vi "Teleop.vi"(10 "Match Info":T1={"Autonomous Elapsed Seconds"=0.0, "TeleOp Elapsed Seconds"=0.0, "Disabled Elapsed Seconds"=0.0, "Visited Autonomous"=FALSE, "Visited TeleOp"=FALSE, "Visited Disabled"=FALSE, "Autonomous Settings"={"Autonomous Style"=enum."Independent", "VI Refnum"=refnum}}, 11 "Call Context":T2) -> ()   [LabVIEW 2015]
doc: "This VI is called for each TeleOp packet received from the DS where the robot is not disabled. It is often used to read from the joysticks and update I/O or to update setpoints for timed control loops. It should complete and return within 20 milliseconds or it may miss DS packets."
uses:
  <vilib>/Rock Robotics/WPI/DriverStation/WPI_DriverStationDerivedRobotMode.ctl
  <vilib>/Rock Robotics/WPI/DriverStation/WPI_DriverStationMatch Info.ctl
  <vilib>/Rock Robotics/WPI/CAN/TalonSRX/WPI_CANTalonSRX_APIControlMode.ctl
  <vilib>/Rock Robotics/WPI/Solenoid/WPI_SolenoidValue.ctl
  <vilib>/Rock Robotics/WPI/Utilities/WPI_GetSetVariantRefNum.vi
  <vilib>/Rock Robotics/Network Tables/NT Read Number.vi
  <vilib>/Rock Robotics/Network Tables/NT Write Boolean.vi
  <vilib>/Rock Robotics/WPI/Solenoid/WPI_SolenoidSetEnum.vi
  <vilib>/Rock Robotics/Network Tables/NT Write Number.vi
  <vilib>/addons/control/pid/NI_PID_pid.lvlib
  <vilib>/addons/control/pid/pid.llb/PID (DBL).vi
  <vilib>/Rock Robotics/WPI/Ultrasonic/WPI_SonarMB1010AnalogRefNum Registry Get.vi
  <vilib>/Rock Robotics/WPI/Ultrasonic/WPI_SonarMB1010AnalogGetRange.vi
panel:
  out "right encoder":dbl
  out "left encoder":dbl
  out "Numeric":dbl
  out "Angular Rate":dbl
  out "Angle":dbl
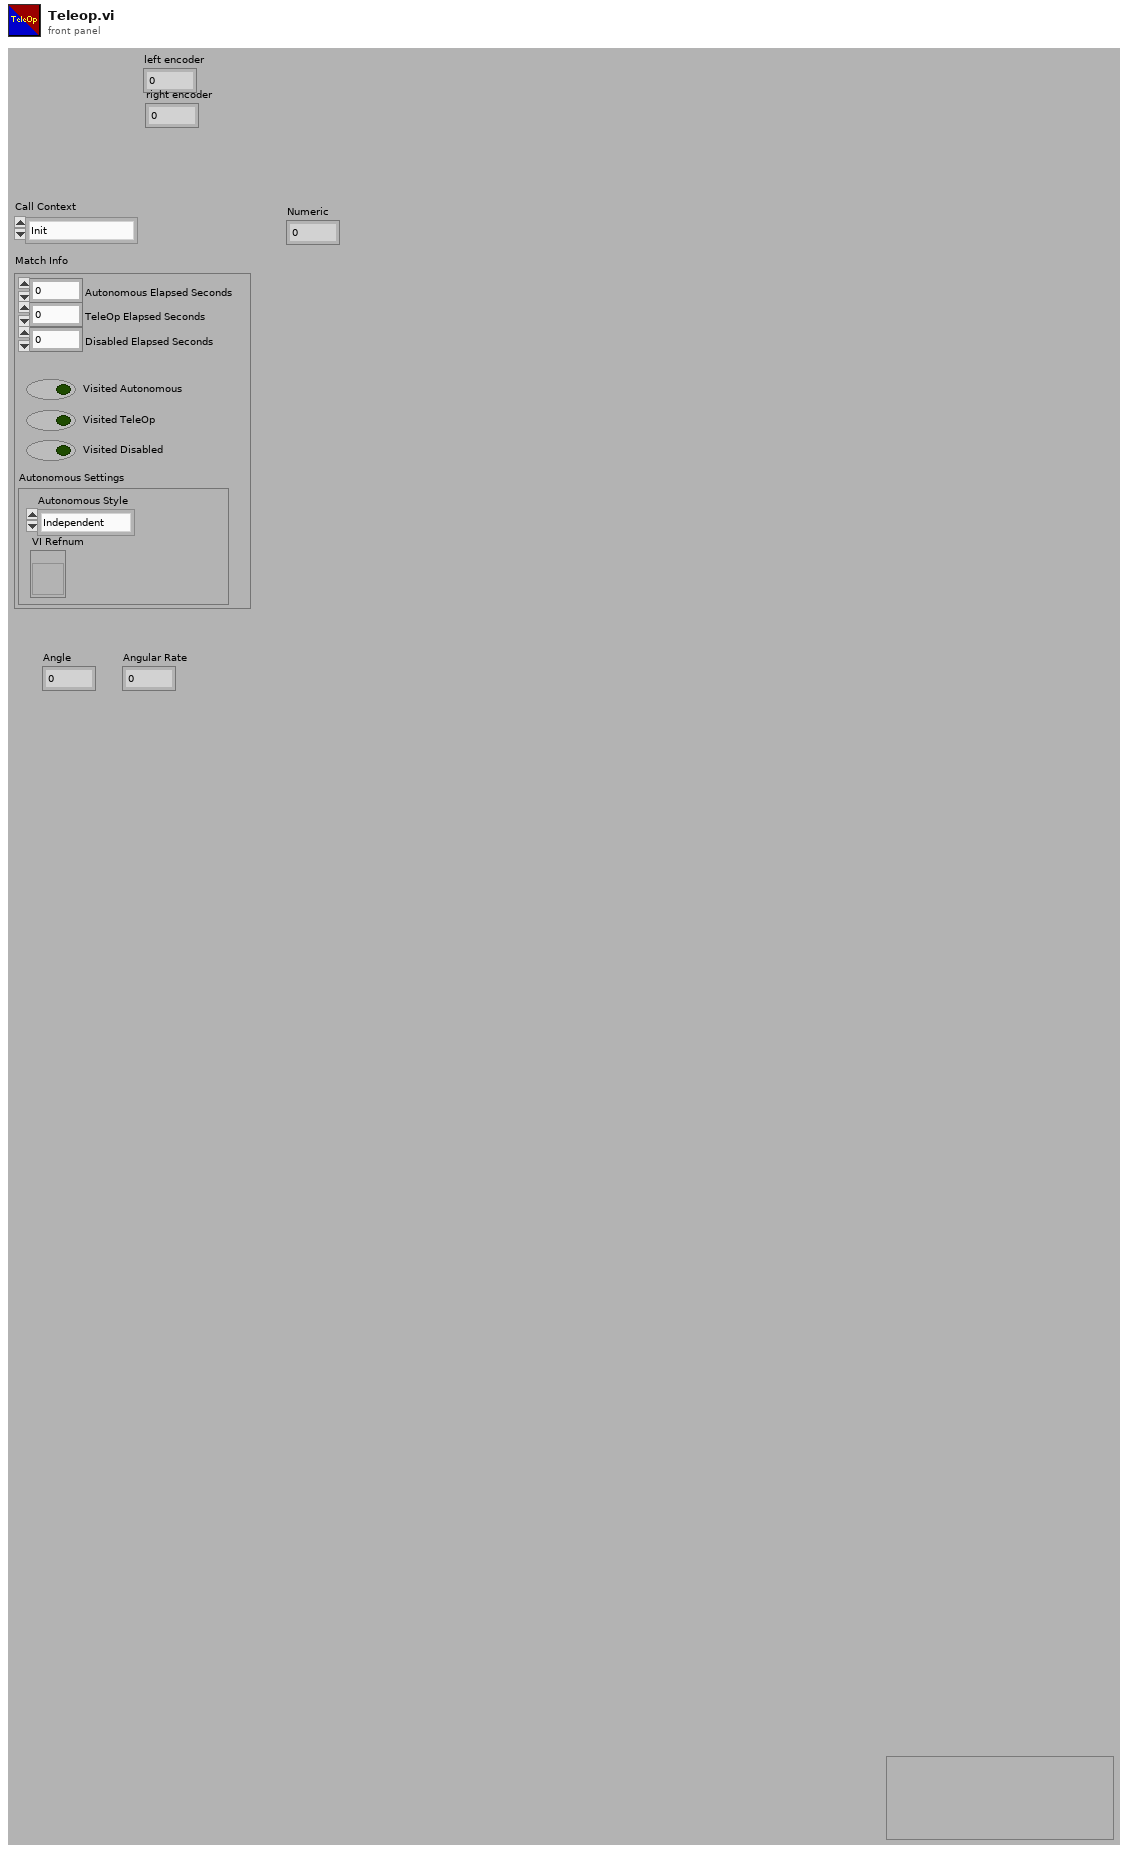
[diagram p1: front panel]
types:
  T1 = typedef "WPI_DriverStationMatch Info.ctl" = cluster{"Autonomous Elapsed Seconds":dbl, "TeleOp Elapsed Seconds":dbl, "Disabled Elapsed Seconds":dbl, "Visited Autonomous":bool, "Visited TeleOp":bool, "Visited Disabled":bool, "Autonomous Settings":cluster{"Autonomous Style":enum16{"Iterative", "Independent"}, "VI Refnum":refnum<vi>}}
  T2 = typedef "WPI_DriverStationDerivedRobotMode.ctl" = enum16{"Init", "Execute", "Stop"}
  T3 = typedef "WPI_JoystickDevRef.ctl" = cluster{"Device":T4}
  T4 = typedef "WPI_JoystickDeviceEnum.ctl" = enum16{"USB 0", "USB 1", "USB 2", "USB 3", "USB 4", "USB 5"}
  T5 = typedef "WPI_CANTalonSRX_APIControlMode.ctl" = enum8{"Percent VBus", "Speed", "Position", "Slave", "Unchanged / Invalid", "Voltage Compensation", "Current", "Motion Profile"}
  T6 = typedef "WPI_SolenoidValue.ctl" = enum16{"Off", "On", "Forward", "Reverse"}
  T7 = typedef "WPI_GyroDevRef.ctl" = cluster{"DevStatus":errorcluster, "Analog Channel":T8, "Offset":dbl, "Gain (VoltsPerDegree/Second)":dbl, "Gyro Type":enum16{"Analog", "XRS450"}, "Handle":i32, "SPI Bus":T9, "Device Found":bool, "Sample Rate":dbl, "Calibrate On Open":bool}
  T8 = typedef "FPGA_AIChannel.ctl" = enum8{"AI 0", "AI 1", "AI 2", "AI 3", "AI MXP 0", "AI MXP 1", "AI MXP 2", "AI MXP 3", "Invalid"}
  T9 = typedef "spi_bus.ctl" = enum16{"SPI On-Board, CS0", "SPI On-Board, CS1", "SPI On-Board, CS2", "SPI On-Board, CS3", "SPI MXP", "Invalid"}
  T10 = typedef "WPI_MotorControlDeviceRef.ctl" = cluster{"DeviceStatus":errorcluster, "Type":T11, "PWM":cluster{"PWM Channel":T12, "DeadBand":T13}, "CAN":cluster{"Device Number":u8, "Control Mode":T14, "Semaphore":T15, "Max Vout":dbl, "TalonSRX Control Mode":T5}, "Invert":bool}
  T11 = typedef "WPI_MotorControlType.ctl" = enum16{"PWM", "CAN", "CANTalonSRX"}
  T12 = typedef "FPGA_DIOPWMChannel.ctl" = enum8{"PWM 0", "PWM 1", "PWM 2", "PWM 3", "PWM 4", "PWM 5", "PWM 6", "PWM 7", "PWM 8", "PWM 9", "PWM MXP 0", "PWM MXP 1", "PWM MXP 2", "PWM MXP 3", "PWM MXP 4", "PWM MXP 5", "PWM MXP 6", "PWM MXP 7", "PWM MXP 8", "PWM MXP 9", "Invalid"}
  T13 = typedef "WPI_PWMDeadband.ctl" = cluster{"Name":string, "maxPositivePwm":i32, "minPositivePwm":i32, "centerPwm":i32, "maxNegativePwm":i32, "minNegativePwm":i32, "angularRange":u16}
  T14 = typedef "WPI_CANJaguar_ControlMode.ctl" = enum8{"Percent VBus", "Current", "Speed", "Position", "Voltage"}
  T15 = typedef "Semaphore RefNum" = refnum<k1>
  T16 = typedef "WPI_ServoDeviceRef.ctl" = cluster{"DeviceStatus":errorcluster, "PWM Channel":T12, "DeadBand":T13}
  T17 = typedef "WPI_CANTalonSRX_GlobalStatus.ctl" = cluster{"Applied Throttle":dbl, "Module Enabled":bool, "CAN Error":errorcluster, "Closed Loop Error":dbl, "Forward Limit Switch Closed":bool, "Reverse Limit Switch Closed":bool, "Sensor Position":dbl, "Sensor Velocity":dbl, "Current":dbl, "Sticky Fault - Over Temp":bool, "Sticky Fault - Under Voltage":bool, "Sticky Fault - Forward Limit":bool, "Sticky Fault - Reverse Limit":bool, "Sticky Fault - Forward Soft Limit":bool, "Sticky Fault - Reverse Soft Limit":bool, "Brake is Enabled":bool, "Encoder Position":dbl, "Encoder Velocity":dbl, "Encoder Index Count":dbl, "Encoder A Pin State":bool, "Encoder B Pin State":bool, "Encoder Index Pin State":bool, "Analog In":dbl, "Analog In Velocity":dbl, "Temperature (C)":dbl, "Battery Voltage":dbl, "Control 5 Is Supported":bool, "Current Profile Slot Select":dbl, "Pos Div 8":bool, "Vel Div 4":bool, "Pulse Width Position":i32, "Pulse Width Velocity":i32, "Pulse Width Rise To Rise (us)":i32, "Pulse Width Rise To Fall (us)":i32, "Mot Prof Active Is Under Run":bool, "Mot Prof Active Has Under Run":bool, "Mot Prof Active Is Last":bool, "Mot Prof Active Velocity Only":bool, "Mot Prof Active Is Valid":bool, "Mot Prof Buffer Is Full":bool, "Mot Prof Active Profile Slot Select":i32, "Mot Prof NextID":i32, "Mot Prof Count":i32, "Mot Prof Active Velocity":dbl, "Mot Prof Active Position":dbl, "Mot Prof Output Enable":i32}
  T18 = typedef "WPI_SonarMB1010AnalogDeviceRef.ctl" = cluster{"AIDeviceRef":T19, "Scaling factor (V/in)":dbl, "Average Bits":u8}
  T19 = typedef "WPI_AnalogChannelDevRef.ctl" = cluster{"DevStatus":errorcluster, "Analog Channel":T8}
  T20 = typedef "WPI_SolenoidDevRef.ctl" = cluster{"DevStatus":errorcluster, "Pneumatics Control Module":u8, "Forward Solenoid Channel":T21, "Reverse Solenoid Channel":T21}
  T21 = typedef "WPI_SolenoidChannel.ctl" = enum8{"Solenoid 0", "Solenoid 1", "Solenoid 2", "Solenoid 3", "Solenoid 4", "Solenoid 5", "Solenoid 6", "Solenoid 7", "Invalid"}
  T22 = cluster{"proportional gain (Kc)":dbl, "integral time (Ti, min)":dbl, "derivative time (Td, min)":dbl}
  T23 = typedef "WPI_PotentiometerDevRef.ctl" = cluster{"DevStatus":errorcluster, "Analog Channel":T8, "Invert Output":bool}
  T24 = cluster{"Aiming?":bool, "X setpoint":dbl, "Y-setpoint":dbl}
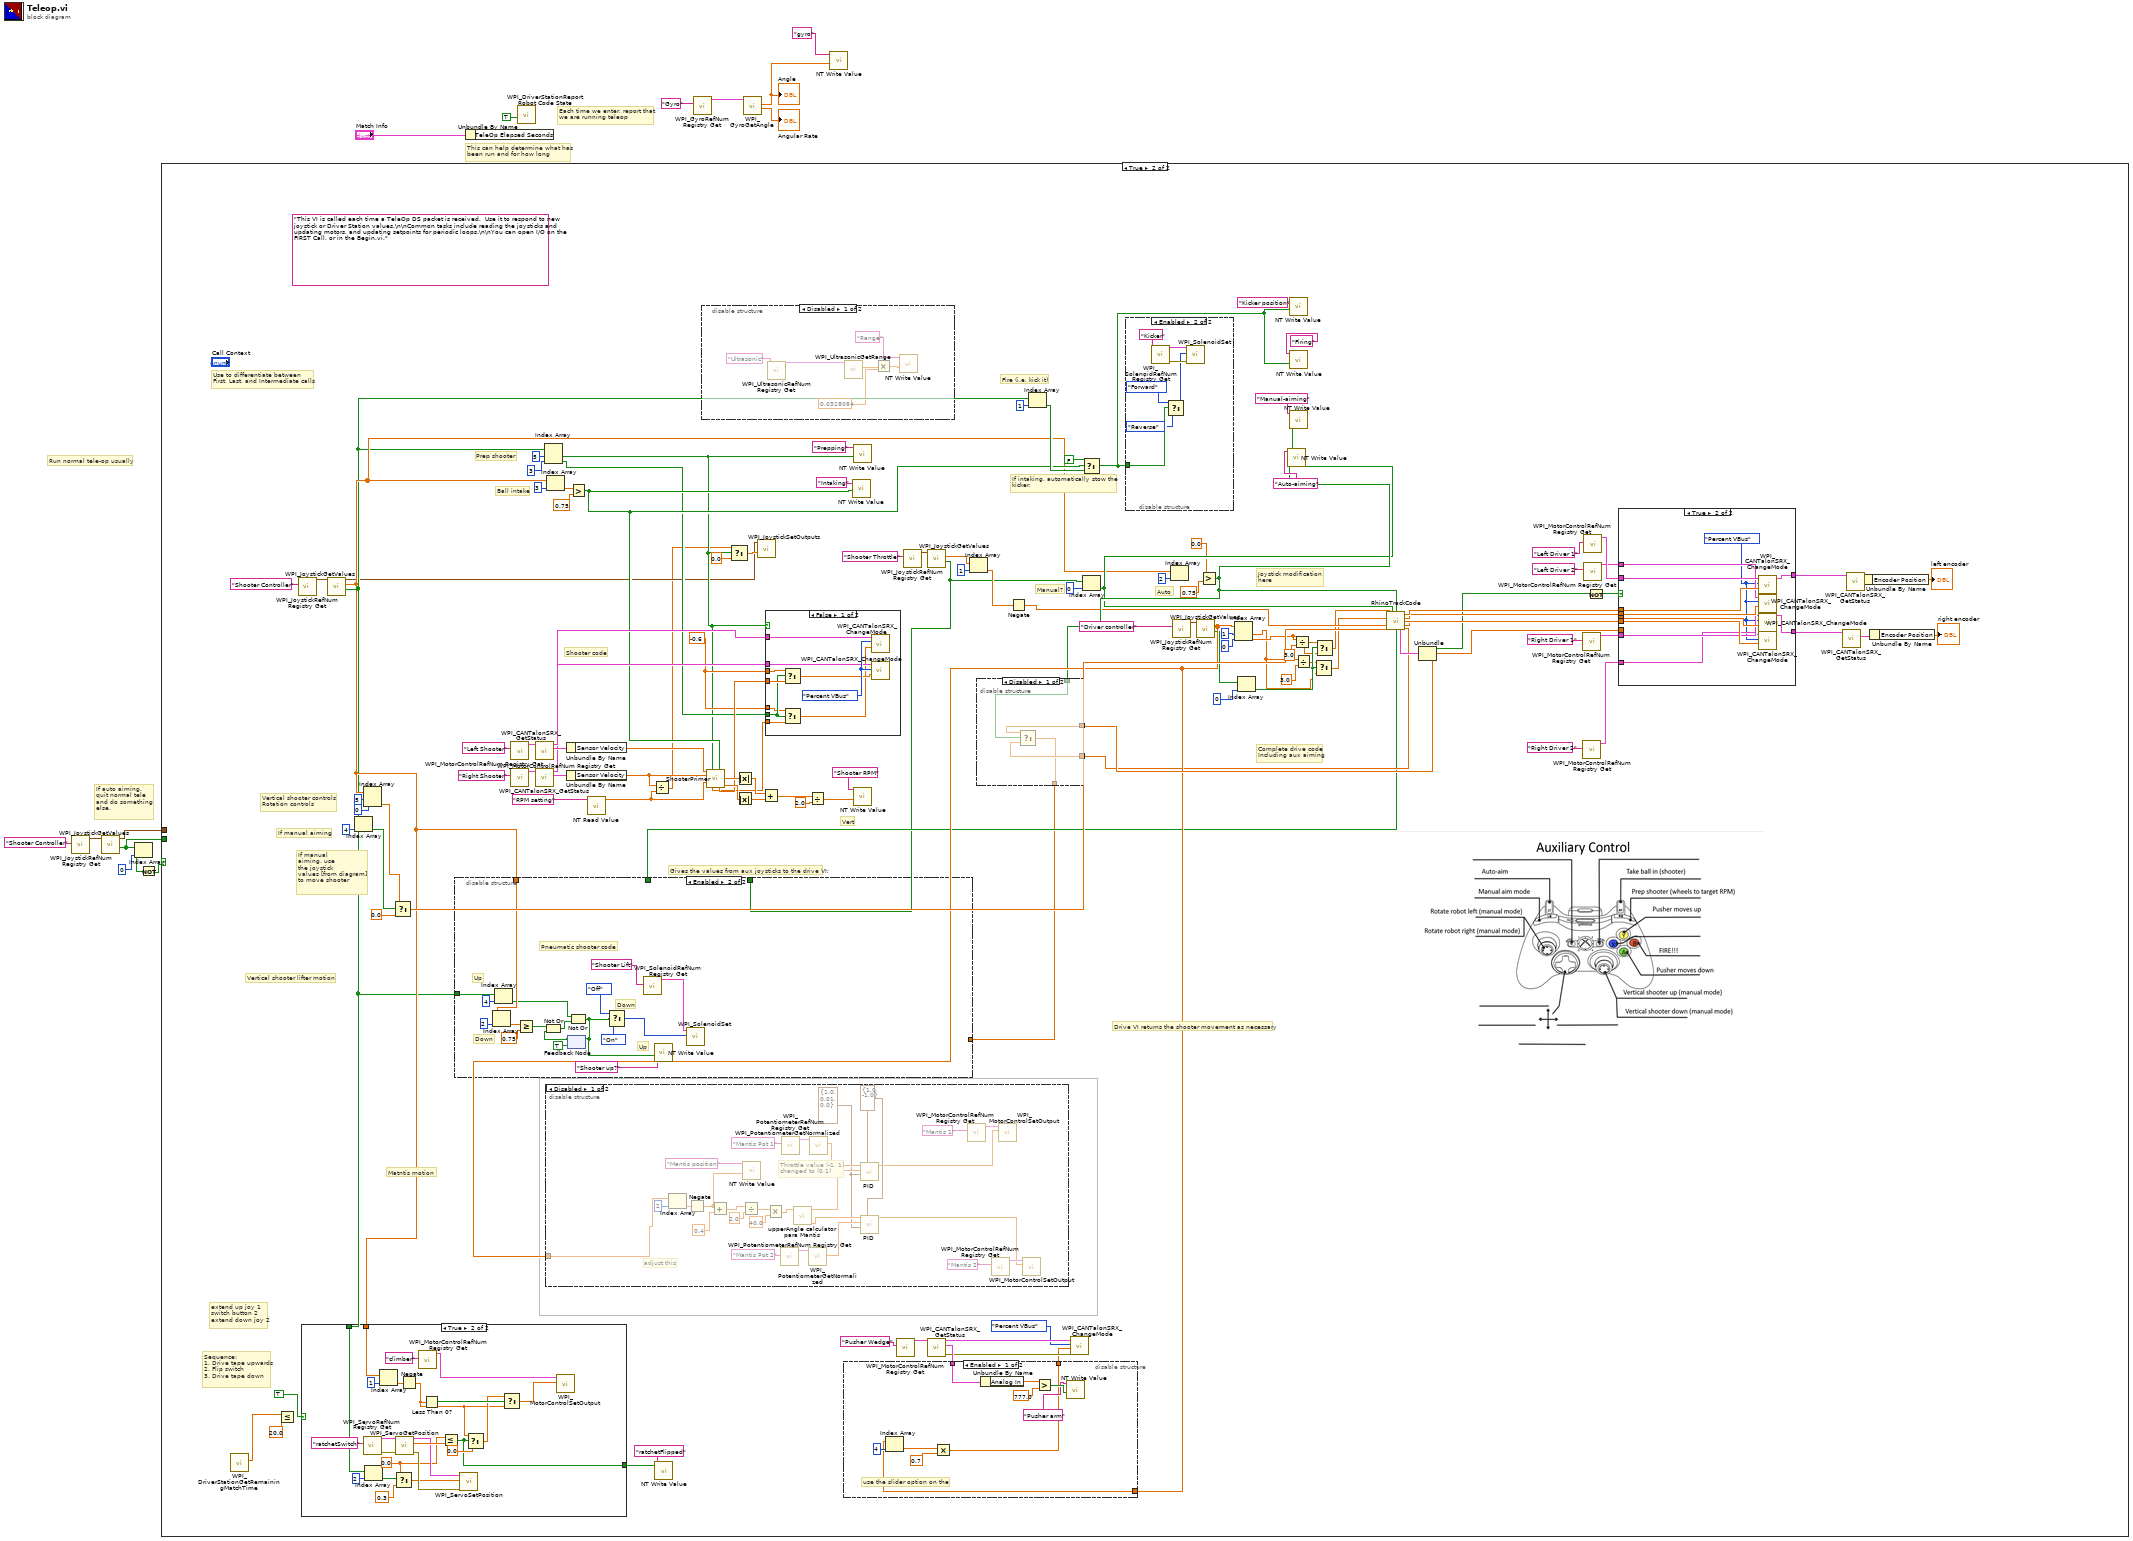
[diagram p0: block diagram]
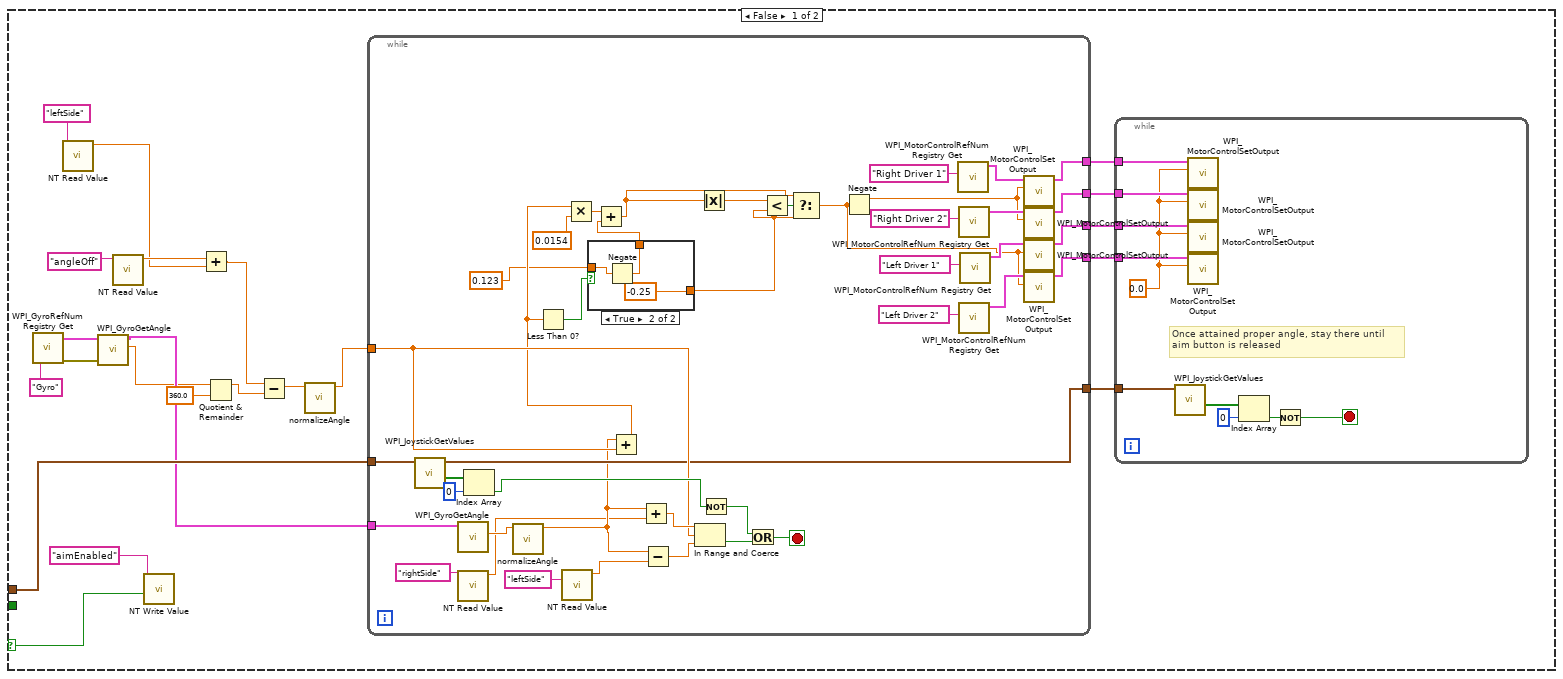
[diagram p2: hidden frame]
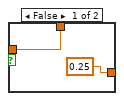
[diagram p3: hidden frame]
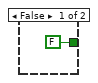
[diagram p4: hidden frame]
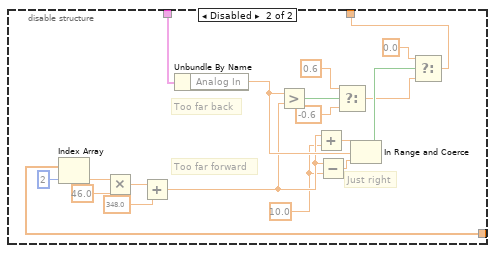
[diagram p5: hidden frame]
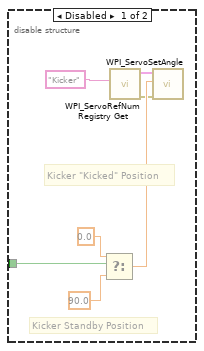
[diagram p6: hidden frame]
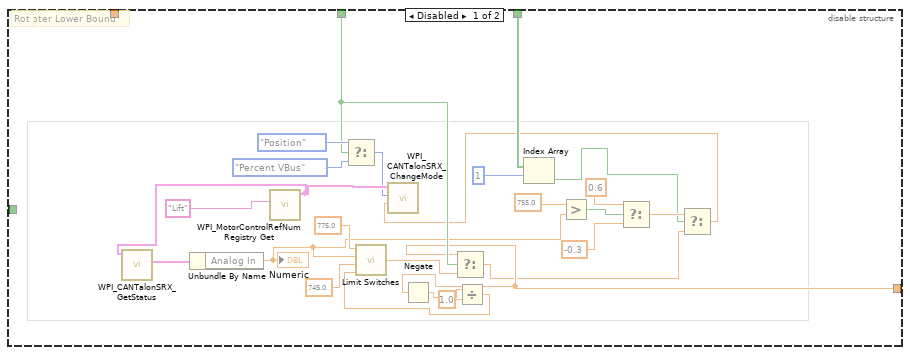
[diagram p8: hidden frame]
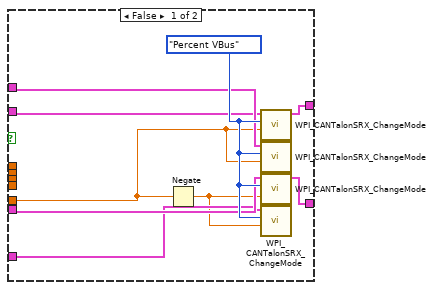
[diagram p10: hidden frame]
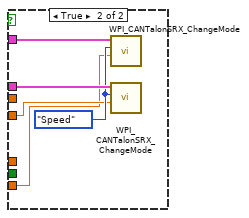
[diagram p11: hidden frame]
diagram:
  # "If auto aiming,\nquit normal tele\nand do something\nelse,"
  # "Run normal tele-op usually"
  # "This can help determine what has\nbeen run and for how long"
  # "Each time we enter, report that\nwe are running teleop"
  n1 = call <vilib>:"WPI_JoystickRefNum Registry Get.vi"("refnum name"="Shooter Controller") -> ("JoystickDevRef"=w11:T3)  [unwired: 9 in, 1 out]
  n2 = call <vilib>:"WPI_JoystickGetValues.vi"("JoystickDevRef"=w11) -> ("Buttons"=w8:bool[], "JoystickDevRef"=w1:T3)  [unwired: 6 in, 3 out]
  n3 = Index Array(array=w8, index=0) -> (element=w9:bool)
  n4 = Not(x=w9) -> (.not. x?=w7:bool)
  n5 = case shown="True" w7 {
    selector: w7 -> [w35 _]
    tunnel: w8 -> [_ _]
    tunnel: w1 -> [w33 _]
    frame False {
      n6 = call <vilib>:"WPI_GyroRefNum Registry Get.vi"("refnum name"="Gyro") -> ("error out"=w24:errorcluster, "GyroDevRef"=w25:T7)  [unwired: 9 in]
      n7 = call-poly <vilib>:"NT Read Value.vi"("Name"="leftSide") -> ("Numeric"=w16:dbl)  [unwired: 9 in, 1 out]
      n8 = call <vilib>:"WPI_GyroGetAngle.vi"("error in"=w24, "GyroDevRef"=w25) -> ("Angle"=w23:dbl, "GyroDevRef"=w26:T7)  [unwired: 5 in, 3 out]
      n9 = call-poly <vilib>:"NT Read Value.vi"("Name"="angleOff") -> ("Numeric"=w18:dbl)  [unwired: 9 in, 1 out]
      n10 = call-poly <vilib>:"NT Write Value.vi"("Boolean"=w35, "Name"="aimEnabled") -> ()  [unwired: 9 in, 1 out]
      n11 = Add(x=w18, y=w16) -> (x+y=w17:dbl)
      n12 = Quotient & Remainder(x=w23, y=360.0) -> (x-y*floor(x/y)=w21:dbl)  [unwired: 1 out]
      n13 = Subtract(x=w17, y=w21) -> (x-y=w20:dbl)
      n14 = call "normalizeAngle.vi"("Input"=w20) -> ("Output"=w19:dbl)  [unwired: 10 in]
      n15 = while {
        tunnel: w33 -> [w80]
        tunnel: w26 -> [w77]
        tunnel: w19 -> [w70]
        tunnel: [w69] -> w31
        tunnel: [w68] -> w30
        tunnel: [w67] -> w29
        tunnel: [w66] -> w28
        tunnel: [w65] -> w27
        stop <- w71 stop-if-true
        n16 = call <vilib>:"WPI_JoystickGetValues.vi"("JoystickDevRef"=w80) -> ("Buttons"=w79:bool[], "JoystickDevRef"=w65:T3)  [unwired: 6 in, 3 out]
        n17 = call <vilib>:"WPI_GyroGetAngle.vi"("GyroDevRef"=w77) -> ("Angle"=w62:dbl)  [unwired: 6 in, 4 out]
        n18 = call-poly <vilib>:"NT Read Value.vi"("Name"="rightSide") -> ("Numeric"=w49:dbl)  [unwired: 9 in, 1 out]
        n19 = Index Array(array=w79, index=0) -> (element=w72:bool)
        n20 = call "normalizeAngle.vi"("Input"=w62) -> ("Output"=w61:dbl)  [unwired: 10 in]
        n21 = call-poly <vilib>:"NT Read Value.vi"("Name"="leftSide") -> ("Numeric"=w50:dbl)  [unwired: 9 in, 1 out]
        n22 = Add(x=w61, y=w70) -> (x+y=w60:dbl)
        n23 = Less Than 0?(x=w60) -> (x < 0?=w54:bool)
        n24 = Multiply(x=w60, y=0.0154) -> (x*y=w58:dbl)
        n25 = case shown="True" w54 {
          tunnel: 0.123 ("y") -> [w90 w93]
          tunnel: [w90 w92] -> w52
          tunnel: [0.25 ("y") -0.25 ("y")] -> w51
          frame False {
          }
          frame True {
            n26 = Negate(x=w93) -> (-x=w92:dbl)
          }
        }
        n27 = Add(x=w58, y=w52) -> (x+y=w56:dbl)
        n28 = Add(x=w61, y=w49) -> (x+y=w76:dbl)
        n29 = Subtract(x=w61, y=w50) -> (x-y=w75:dbl)
        n30 = In Range and Coerce(upper limit=w76, x=w70, lower limit=w75) -> (In Range?=w74:bool)  [unwired: 1 out]
        n31 = Absolute Value(x=w56) -> (abs(x)=w55:dbl)
        n32 = Not(x=w72) -> (.not. x?=w73:bool)
        n33 = Or(x=w73, y=w74) -> (x .or. y?=w71:bool)
        n34 = Less?(x=w55, y=w51) -> (x < y?=w57:bool)
        n35 = Select(t=w56, s=w57, f=w51) -> (s? t:f=w64:dbl)
        n36 = Negate(x=w64) -> (-x=w63:dbl)
        n37 = call <vilib>:"WPI_MotorControlRefNum Registry Get.vi"("refnum name"="Right Driver 1") -> ("MotorControlDevRef"=w84:T10)  [unwired: 9 in, 1 out]
        n38 = call <vilib>:"WPI_MotorControlRefNum Registry Get.vi"("refnum name"="Right Driver 2") -> ("MotorControlDevRef"=w83:T10)  [unwired: 9 in, 1 out]
        n39 = call <vilib>:"WPI_MotorControlRefNum Registry Get.vi"("refnum name"="Left Driver 2") -> ("MotorControlDevRef"=w81:T10)  [unwired: 9 in, 1 out]
        n40 = call <vilib>:"WPI_MotorControlRefNum Registry Get.vi"("refnum name"="Left Driver 1") -> ("MotorControlDevRef"=w82:T10)  [unwired: 9 in, 1 out]
        n41 = call <vilib>:"WPI_MotorControlSetOutput.vi"("Output"=w63, "MotorControlDevRef"=w84) -> ("MotorControlDevRef"=w69:T10)  [unwired: 7 in, 2 out]
        n42 = call <vilib>:"WPI_MotorControlSetOutput.vi"("Output"=w63, "MotorControlDevRef"=w83) -> ("MotorControlDevRef"=w68:T10)  [unwired: 7 in, 2 out]
        n43 = call <vilib>:"WPI_MotorControlSetOutput.vi"("Output"=w64, "MotorControlDevRef"=w82) -> ("MotorControlDevRef"=w67:T10)  [unwired: 7 in, 2 out]
        n44 = call <vilib>:"WPI_MotorControlSetOutput.vi"("Output"=w64, "MotorControlDevRef"=w81) -> ("MotorControlDevRef"=w66:T10)  [unwired: 7 in, 2 out]
      }
      n45 = while {
        tunnel: w31 -> [w46]
        tunnel: w30 -> [w45]
        tunnel: w29 -> [w44]
        tunnel: w28 -> [w43]
        tunnel: w27 -> [w41]
        stop <- w37 stop-if-true
        w42 = 0.0
        # "Once attained proper angle, stay there until \naim button is released"
        n46 = call <vilib>:"WPI_JoystickGetValues.vi"("JoystickDevRef"=w41) -> ("Buttons"=w40:bool[])  [unwired: 6 in, 4 out]
        n47 = call <vilib>:"WPI_MotorControlSetOutput.vi"("Output"=w42, "MotorControlDevRef"=w46) -> ()  [unwired: 7 in, 3 out]
        n48 = call <vilib>:"WPI_MotorControlSetOutput.vi"("Output"=w42, "MotorControlDevRef"=w45) -> ()  [unwired: 7 in, 3 out]
        n49 = call <vilib>:"WPI_MotorControlSetOutput.vi"("Output"=w42, "MotorControlDevRef"=w44) -> ()  [unwired: 7 in, 3 out]
        n50 = call <vilib>:"WPI_MotorControlSetOutput.vi"("Output"=w42, "MotorControlDevRef"=w43) -> ()  [unwired: 7 in, 3 out]
        n51 = Index Array(array=w40, index=0) -> (element=w38:bool)
        n52 = Not(x=w38) -> (.not. x?=w37:bool)
      }
    }
    frame True {
      w127 = -0.6
      (unwired) "This VI is called each time a TeleOp DS packet is received.  Use it to respond to new joystick or Driver Station values.\n\nCommon tasks include reading the joysticks and updating motors, and updating setpoints for periodic loops.\n\nYou can open I/O on the FIRST Call, or in the Begin.vi."
      # "extend up joy 1\nswitch button 2\nextend down joy 2"
      # "Sequence:\n1. Drive tape upwards\n2. Flip switch\n3. Drive tape down"
      # "Auto"
      # "Manual?"
      # "Joystick modification\nhere"
      # "Complete drive code\nIncluding aux aiming"
      # "If intaking, automatically stow the\nkicker,"
      # "Fire (i.e, kick it)"
      # "Shooter code"
      # "Drive VI returns the shooter movement as necessary"
      # "Gives the values from aux joysticks to the drive VI;"
      # "Vert"
      # "If manual \naiming, use\nthe joystick\nvalues [from diagram]\nto move shooter"
      # "Vertical shooter controls\nRotation controls"
      # "If manual aiming"
      # "Ball intake"
      # "Prep shooter"
      # "Matntis motion"
      # "Vertical shooter lifter motion"
      # "Use to differentiate between\nFirst, Last, and Intermediate calls"
      n53 = call <vilib>:"WPI_DriverStationGetRemainingMatchTime.vi"() -> ("Match Time(s)"=w110:sgl)  [unwired: 10 in, 1 out]
      n54 = Less Or Equal?(x=w110, y=20.0) -> ()  [unwired: 1 out]
      n55 = call <vilib>:"WPI_JoystickRefNum Registry Get.vi"("refnum name"="Shooter Controller") -> ("JoystickDevRef"=w215:T3)  [unwired: 9 in, 1 out]
      n56 = call <vilib>:"WPI_JoystickGetValues.vi"("JoystickDevRef"=w215) -> ("Buttons"=w112:bool[], "Axes"=w113:dbl[], "JoystickDevRef"=w103:T3)  [unwired: 6 in, 2 out]
      n57 = case shown="True" TRUE {
        tunnel: w113 -> [_ w240]
        tunnel: w112 -> [_ w239]
        tunnel: [FALSE w218] -> w108
        frame False {
        }
        frame True {
          w219 = 0.0 ("t")
          n58 = call <vilib>:"WPI_ServoRefNum Registry Get.vi"("refnum name"="ratchetSwitch") -> ("error out"=w232:errorcluster, "ServoDeviceRef"=w233:T16)  [unwired: 9 in]
          n59 = Index Array(array=w239, index=2) -> (element=w221:bool)
          n60 = Index Array(array=w240, index=1) -> (element=w230:dbl)
          n61 = Select(t=w219, s=w221, f=0.3) -> (s? t:f=w222:dbl)
          n62 = call <vilib>:"WPI_ServoGetPosition.vi"("error in (no error)"=w232, "ServoDeviceRef"=w233) -> ("error out"=w223:errorcluster, "Position"=w229:dbl, "ServoDeviceRef"=w224:T16)  [unwired: 7 in]
          n63 = Negate(x=w230) -> (-x=w226:dbl)
          n64 = call <vilib>:"WPI_MotorControlRefNum Registry Get.vi"("refnum name"="climber") -> ("MotorControlDevRef"=w234:T10)  [unwired: 9 in, 1 out]
          n65 = Less Than 0?(x=w226) -> (x < 0?=w231:bool)
          n66 = Less Or Equal?(x=w219, y=w229) -> (x <= y?=w218:bool)
          n67 = call <vilib>:"WPI_ServoSetPosition.vi"("error in (no error)"=w223, "Position"=w222, "ServoDeviceRef"=w224) -> ()  [unwired: 7 in, 2 out]
          n68 = Select(t=w226, s=w218, f=0.0) -> (s? t:f=w228:dbl)
          n69 = Select(t=w228, s=w231, f=w226) -> (s? t:f=w225:dbl)
          n70 = call <vilib>:"WPI_MotorControlSetOutput.vi"("Output"=w225, "MotorControlDevRef"=w234) -> ()  [unwired: 7 in, 3 out]
        }
      }
      n71 = Index Array(array=w112, index=4) -> (element=w203:bool)
      n72 = Index Array(array=w113, index #1=5 ("index"), index #2=0 ("index")) -> (element #2=w205:dbl)  [unwired: 1 out]
      n73 = Select(t=w205, s=w203, f=0.0) -> (s? t:f=w204:dbl)
      n74 = call <vilib>:"WPI_MotorControlRefNum Registry Get.vi"("refnum name"="Left Shooter") -> ("MotorControlDevRef"=w190:T10)  [unwired: 9 in, 1 out]
      n75 = call <vilib>:"WPI_MotorControlRefNum Registry Get.vi"("refnum name"="Right Shooter") -> ("MotorControlDevRef"=w191:T10)  [unwired: 9 in, 1 out]
      n76 = call <vilib>:"WPI_CANTalonSRX_GetStatus.vi"("CAN Talon SRX Ref"=w190) -> ("Talon SRX Status"=w180:T17, "CAN Talon SRX Ref"=w178:T10)  [unwired: 8 in, 1 out]
      n77 = call <vilib>:"WPI_CANTalonSRX_GetStatus.vi"("CAN Talon SRX Ref"=w191) -> ("Talon SRX Status"=w181:T17, "CAN Talon SRX Ref"=w177:T10)  [unwired: 8 in, 1 out]
      n78 = Index Array(array=w112, index #1=5 ("index"), index #2=3 ("index")) -> (element #1=w105:bool, element #2=w115:bool)
      n79 = Index Array(array=w113, index=3) -> (element=w210:dbl)
      n80 = Unbundle By Name(w180) -> ("Sensor Velocity"=w179:dbl)
      n81 = Unbundle By Name(w181) -> ("Sensor Velocity"=w102:dbl)
      n82 = Greater?(x=w210, y=0.75) -> (0:w116:bool)
      n83 = call-poly <vilib>:"NT Read Value.vi"("Name"="RPM setting") -> ("Numeric"=w101:dbl)  [unwired: 9 in, 1 out]
      n84 = Divide(x=w102, y=w101) -> (x/y=w100:dbl)
      n85 = call-poly <vilib>:"NT Write Value.vi"("Boolean"=w108, "Name"="ratchetFlipped") -> ()  [unwired: 9 in, 1 out]
      n86 = disable-structure shown="Disabled" {
        frame Disabled {
          n87 = call-poly <vilib>:"WPI_UltrasonicRefNum Registry Get.vi"("refnum name"="Ultrasonic") -> ("SonarMB1010AnalogDevRef"=w335:T18)  [unwired: 9 in, 1 out]
          n88 = call-poly <vilib>:"WPI_UltrasonicGetRange.vi"("SonarMB1010AnalogDevRef"=w335) -> ("Distance"=w333:dbl)  [unwired: 8 in, 2 out]
          n89 = Multiply(x=w333, y=0.0328084) -> (x*y=w332:dbl)
          n90 = call-poly <vilib>:"NT Write Value.vi"("Numeric"=w332, "Name"="Range") -> ()  [unwired: 9 in, 1 out]
        }
        frame Enabled {
        }
      }
      n91 = call "ShooterPrimer.vi"("Left RPM"=w179, "Shooter Prime"=w105, "Intake Mode"=w116, "Right RPM"=w102, "Desired RPM"=w101) -> ("Left RPM"=w183:dbl, "Left Motor Output"=w175:dbl, "Right Motor Output"=w176:dbl, "Right RPM"=w182:dbl)  [unwired: 7 in]
      n92 = Select(t=w100, s=w105, f=0.0) -> (s? t:f=w106:dbl)
      n93 = Absolute Value(x=w183) -> (abs(x)=w185:dbl)
      n94 = Absolute Value(x=w182) -> (abs(x)=w184:dbl)
      n95 = call <vilib>:"WPI_JoystickSetOutputs.vi"("Right Rumble"=w106, "JoystickDevRef"=w103) -> ()  [unwired: 8 in, 2 out]
      n96 = Add(x=w185, y=w184) -> (x+y=w187:dbl)
      n97 = case shown="False" w105 {
        tunnel: w178 -> [w365 w371]
        tunnel: w177 -> [w364 w370]
        tunnel: w176 -> [w362 w368]
        tunnel: w175 -> [w363 w367]
        tunnel: w115 -> [w361 _]
        tunnel: w127 -> [w358 _]
        tunnel: w127 -> [w357 _]
        frame False {
          w366 = WPI_CANTalonSRX_APIControlMode."Percent VBus" ("Control Mode")
          n98 = Select(t=w358, s=w361, f=w362) -> (s? t:f=w360:dbl)
          n99 = Select(t=w357, s=w361, f=w363) -> (s? t:f=w359:dbl)
          n100 = call <vilib>:"WPI_CANTalonSRX_ChangeMode.vi"("Output"=w359, "Control Mode"=w366, "CAN Talon SRX Ref"=w364) -> ()  [unwired: 7 in, 2 out]
          n101 = call <vilib>:"WPI_CANTalonSRX_ChangeMode.vi"("Output"=w360, "Control Mode"=w366, "CAN Talon SRX Ref"=w365) -> ()  [unwired: 7 in, 2 out]
        }
        frame True {
          w369 = WPI_CANTalonSRX_APIControlMode."Speed" ("Control Mode")
          n102 = call <vilib>:"WPI_CANTalonSRX_ChangeMode.vi"("Output"=w367, "Control Mode"=w369, "CAN Talon SRX Ref"=w370) -> ()  [unwired: 7 in, 2 out]
          n103 = call <vilib>:"WPI_CANTalonSRX_ChangeMode.vi"("Output"=w368, "Control Mode"=w369, "CAN Talon SRX Ref"=w371) -> ()  [unwired: 7 in, 2 out]
        }
      }
      n104 = Divide(x=w187, y=2.0) -> (x/y=w195:dbl)
      n105 = call-poly <vilib>:"NT Write Value.vi"("Boolean"=w116, "Name"="Intaking") -> ()  [unwired: 9 in, 1 out]
      n106 = call-poly <vilib>:"NT Write Value.vi"("Boolean"=w105, "Name"="Prepping") -> ()  [unwired: 9 in, 1 out]
      n107 = call-poly <vilib>:"NT Write Value.vi"("Numeric"=w195, "Name"="Shooter RPM") -> ()  [unwired: 9 in, 1 out]
      n108 = call <vilib>:"WPI_MotorControlRefNum Registry Get.vi"("refnum name"="Pusher Wedge") -> ("MotorControlDevRef"=w132:T10)  [unwired: 9 in, 1 out]
      n109 = call <vilib>:"WPI_JoystickRefNum Registry Get.vi"("refnum name"="Shooter Throttle") -> ("JoystickDevRef"=w145:T3)  [unwired: 9 in, 1 out]
      n110 = call <vilib>:"WPI_JoystickGetValues.vi"("JoystickDevRef"=w145) -> ("Buttons"=w135:bool[], "Axes"=w136:dbl[])  [unwired: 6 in, 3 out]
      n111 = call <vilib>:"WPI_CANTalonSRX_GetStatus.vi"("CAN Talon SRX Ref"=w132) -> ("error out"=w131:errorcluster, "Talon SRX Status"=w147:T17, "CAN Talon SRX Ref"=w130:T10)  [unwired: 8 in]
      n112 = Index Array(array=w136, index=1) -> (element=w143:dbl)
      n113 = Negate(x=w143) -> (-x=w142:dbl)
      n114 = Index Array(array=w112, index=1) -> (element=w192:bool)
      n115 = Select(t=FALSE, s=w116, f=w192) -> (s? t:f=w199:bool)
      n116 = Index Array(array=w135, index=0) -> (element=w139:bool)
      n117 = disable-structure shown="Enabled" {
        disable-tunnel: w199 -> [w276 w281]
        frame Disabled {
          # "Kicker Standby Position"
          # "Kicker \"Kicked\" Position"
          n118 = Select(t=0.0, s=w276, f=90.0) -> (s? t:f=w275:dbl)
          n119 = call <vilib>:"WPI_ServoRefNum Registry Get.vi"("refnum name"="Kicker") -> ("error out"=w270:errorcluster, "ServoDeviceRef"=w271:T16)  [unwired: 9 in]
          n120 = call <vilib>:"WPI_ServoSetAngle.vi"("error in (no error)"=w270, "Angle"=w275, "ServoDeviceRef"=w271) -> ()  [unwired: 7 in, 2 out]
        }
        frame Enabled {
          n121 = call <vilib>:"WPI_SolenoidRefNum Registry Get.vi"("refnum name"="Kicker") -> ("error out"=w283:errorcluster, "SolenoidDevRef"=w282:T20)  [unwired: 9 in]
          n122 = Select(t=WPI_SolenoidValue."Forward" ("Value"), s=w281, f=WPI_SolenoidValue."Reverse" ("Value")) -> (s? t:f=w279:T6)
          n123 = call-poly <vilib>:"WPI_SolenoidSet.vi"("error in (no error)"=w283, "Value"=w279, "SolenoidDevRef"=w282) -> ()  [unwired: 7 in, 2 out]
        }
      }
      n124 = Index Array(array=w113, index=2) -> ()  [unwired: 1 out]
      n125 = call <vilib>:"WPI_JoystickRefNum Registry Get.vi"("refnum name"="Driver controller") -> ("JoystickDevRef"=w173:T3)  [unwired: 9 in, 1 out]
      n126 = call <vilib>:"WPI_JoystickGetValues.vi"("JoystickDevRef"=w173) -> ("Buttons"=w133:bool[], "Axes"=w150:dbl[])  [unwired: 6 in, 3 out]
      n127 = disable-structure shown="Disabled" {
        disable-tunnel: w150 -> [w372 _]
        frame Disabled {
          w382 = cluster{"output high":dbl, "output low":dbl} {"output high"=1.0, "output low"=-1.0} ("output range")
          w383 = T22 {"proportional gain (Kc)"=1.0, "integral time (Ti, min)"=0.01, "derivative time (Td, min)"=0.0} ("PID gains")
          # "adjust this"
          # "Throttle value (-1, 1)\nchanged to (0,1)"
          n128 = Index Array(array=w372, index=2) -> (element=w374:dbl)
          n129 = Negate(x=w374) -> (-x=w373:dbl)
          n130 = Add(x=w373, y=0.4) -> (x+y=w389:dbl)
          n131 = Divide(x=w389, y=2.0) -> (x/y=w379:dbl)
          n132 = call-poly <vilib>:"NT Write Value.vi"("Numeric"=w373, "Name"="Mantis position") -> ()  [unwired: 9 in, 1 out]
          n133 = Multiply(x=w379, y=40.0) -> (x*y=w378:dbl)
          n134 = call <vilib>:"WPI_PotentiometerRefNum Registry Get.vi"("refnum name"="Mantis Pot 2") -> ("PotDevRef"=w390:T23)  [unwired: 9 in, 1 out]
          n135 = call <vilib>:"WPI_PotentiometerRefNum Registry Get.vi"("refnum name"="Mantis Pot 1") -> ("PotDevRef"=w394:T23)  [unwired: 9 in, 1 out]
          n136 = call "upperAngle calculator para Mantis.vi"("Height to reach"=w378) -> ("Lower Angle"=w385:dbl, "Upper Angle"=w386:dbl)  [unwired: 9 in]
          n137 = call <vilib>:"WPI_PotentiometerGetNormalized.vi"("PotDevRef"=w390) -> ("Normalized Value"=w384:dbl)  [unwired: 8 in, 2 out]
          n138 = call <vilib>:"WPI_PotentiometerGetNormalized.vi"("PotDevRef"=w394) -> ("Normalized Value"=w387:dbl)  [unwired: 8 in, 2 out]
          n139 = call-poly <vilib>:"PID.vi"("output range"=w382, "PID gains"=w383, "process variable"=w387, "setpoint"=w386) -> ("output"=w381:dbl)  [unwired: 6 in, 1 out]
          n140 = call-poly <vilib>:"PID.vi"("output range"=w382, "PID gains"=w383, "process variable"=w384, "setpoint"=w385) -> ("output"=w380:dbl)  [unwired: 6 in, 1 out]
          n141 = call <vilib>:"WPI_MotorControlRefNum Registry Get.vi"("refnum name"="Mantis 1") -> ("MotorControlDevRef"=w396:T10)  [unwired: 9 in, 1 out]
          n142 = call <vilib>:"WPI_MotorControlRefNum Registry Get.vi"("refnum name"="Mantis 2") -> ("MotorControlDevRef"=w392:T10)  [unwired: 9 in, 1 out]
          n143 = call <vilib>:"WPI_MotorControlSetOutput.vi"("Output"=w381, "MotorControlDevRef"=w396) -> ()  [unwired: 7 in, 3 out]
          n144 = call <vilib>:"WPI_MotorControlSetOutput.vi"("Output"=w380, "MotorControlDevRef"=w392) -> ()  [unwired: 7 in, 3 out]
        }
        frame Enabled {
        }
      }
      n145 = disable-structure shown="Enabled" {
        disable-tunnel: w150 -> [w247 w269]
        disable-tunnel: w147 -> [w246 w263]
        disable-tunnel: [w241 w255] -> w129
        frame Enabled {
          # "use the slider option on the"
          n146 = Index Array(array=w247, index=4) -> (element=w249:dbl)
          n147 = Multiply(x=w249, y=0.7) -> (x*y=w241:dbl)
          n148 = Unbundle By Name(w246) -> ("Analog In"=w242:dbl)
          n149 = Greater?(x=w242, y=777.0) -> (0:w244:bool)
          n150 = call-poly <vilib>:"NT Write Value.vi"("Boolean"=w244, "Name"="Pusher arm") -> ()  [unwired: 9 in, 1 out]
        }
        frame Disabled {
          w258 = 10.0
          # "Just right"
          # "Too far forward"
          # "Too far back"
          n151 = Index Array(array=w269, index=2) -> (element=w267:dbl)
          n152 = Multiply(x=w267, y=46.0) -> (x*y=w265:dbl)
          n153 = Add(x=w265, y=348.0) -> (x+y=w259:dbl)
          n154 = Unbundle By Name(w263) -> ("Analog In"=w262:dbl)
          n155 = Greater?(x=w262, y=w259) -> (0:w253:bool)
          n156 = Add(x=w259, y=w258) -> (x+y=w261:dbl)
          n157 = Subtract(x=w259, y=w258) -> (x-y=w260:dbl)
          n158 = Select(t=0.6, s=w253, f=-0.6) -> (s? t:f=w254:dbl)
          n159 = In Range and Coerce(upper limit=w261, x=w262, lower limit=w260) -> (In Range?=w257:bool)  [unwired: 1 out]
          n160 = Select(t=0.0, s=w257, f=w254) -> (s? t:f=w255:dbl)
        }
      }
      n161 = call <vilib>:"WPI_CANTalonSRX_ChangeMode.vi"("error in (no error)"=w131, "Output"=w129, "Control Mode"=WPI_CANTalonSRX_APIControlMode."Percent VBus", "CAN Talon SRX Ref"=w130) -> ()  [unwired: 6 in, 2 out]
      n162 = Greater?(x=0.0 ("y"), y=0.75) -> (0:w149:bool)
      n163 = Index Array(array=w150, index #1=1 ("index"), index #2=0 ("index")) -> (element #1=w117:dbl, element #2=w118:dbl)
      n164 = Index Array(array=w133, index=0) -> (element=w125:bool)
      n165 = call-poly <vilib>:"NT Write Value.vi"("Boolean"=w149, "Name"="Auto-aiming") -> ()  [unwired: 9 in, 1 out]
      n166 = call-poly <vilib>:"NT Write Value.vi"("Boolean"=w199, "Name"="Kicker position") -> ()  [unwired: 9 in, 1 out]
      n167 = call-poly <vilib>:"NT Write Value.vi"("Boolean"=w199, "Name"="Firing") -> ()  [unwired: 9 in, 1 out]
      n168 = call-poly <vilib>:"NT Write Value.vi"("Boolean"=w139, "Name"="Manual-aiming") -> ()  [unwired: 9 in, 1 out]
      n169 = Divide(x=w118, y=3.0) -> (x/y=w124:dbl)
      n170 = Divide(x=w117, y=3.0) -> (x/y=w123:dbl)
      n171 = Select(t=w123, s=w125, f=w117) -> (s? t:f=w119:dbl)
      n172 = Select(t=w124, s=w125, f=w118) -> (s? t:f=w120:dbl)
      n173 = call "RhinoTrackCode.vi"("Y Driver Control"=w120, "Manual Aim Mode"=w139, "Auto aimer"=w149, "X Driver Control"=w119, "Shooter Y"=w142, "Shooter X"=w204) -> ("Left Driver 1"=w172:dbl, "Left Driver 2"=w171:dbl, "Right Driver 1"=w170:dbl, "Right Driver 2"=w169:dbl, "Autoaim?"=w141:bool, "Aiming stuff"=w163:T24, "Shooter Y Motion"=w148:dbl)  [unwired: 2 in, 1 out]
      n174 = Unbundle(w163) -> ("Aiming?"=w138:bool, "X setpoint"=w153:dbl, "Y-setpoint"=w152:dbl)
      n175 = disable-structure shown="Disabled" {
        disable-tunnel: w152 -> [w287 _]
        disable-tunnel: w149 -> [w286 _]
        disable-tunnel: w148 -> [w285 _]
        disable-tunnel: [w284 _] -> w140
        frame Disabled {
          n176 = Select(t=w287, s=w286, f=w285) -> (s? t:f=w284:dbl)
        }
        frame Enabled {
        }
      }
      n177 = disable-structure shown="Enabled" {
        disable-tunnel: w141 -> [w306 _]
        disable-tunnel: w140 -> [w305 _]
        disable-tunnel: w135 -> [w290 _]
        disable-tunnel: w112 -> [_ w329]
        disable-tunnel: w113 -> [_ w326]
        frame Disabled {
          # "Shooter Upper Bound"
          # "Shooter Lower Bound"
          # "Rot"
          n178 = call <vilib>:"WPI_MotorControlRefNum Registry Get.vi"("refnum name"="Lift") -> ("MotorControlDevRef"=w310:T10)  [unwired: 9 in, 1 out]
          n179 = call <vilib>:"WPI_CANTalonSRX_GetStatus.vi"("CAN Talon SRX Ref"=w310) -> ("Talon SRX Status"=w311:T17)  [unwired: 8 in, 2 out]
          n180 = Unbundle By Name(w311) -> ("Analog In"=w296:dbl)
          "Numeric" <- w296
          n181 = Select(t=WPI_CANTalonSRX_APIControlMode."Position" ("Control Mode"), s=w306, f=WPI_CANTalonSRX_APIControlMode."Percent VBus" ("Control Mode")) -> (s? t:f=w307:T5)
          n182 = Negate(x=w305) -> (-x=w300:dbl)
          n183 = Divide(x=w300, y=1.0) -> (x/y=w299:dbl)
          n184 = call "Limit Switches.vi"("Desired Motion"=w299, "Lower Bound"=745.0 ("Upper Bound"), "Input"=w296, "Upper Bound"=775.0) -> ("Allowed Motion"=w302:dbl)
          n185 = Select(t=w305, s=w306, f=w302) -> (s? t:f=w289:dbl)
          n186 = Index Array(array=w290, index=1) -> (element=w291:bool)
          n187 = Greater?(x=755.0 ("Upper Bound"), y=w296) -> (0:w295:bool)
          n188 = Select(t=0.6, s=w295, f=-0.3) -> (s? t:f=w292:dbl)
          n189 = Select(t=w292, s=w291, f=w289) -> (s? t:f=w288:dbl)
          n190 = call <vilib>:"WPI_CANTalonSRX_ChangeMode.vi"("Output"=w288, "Control Mode"=w307, "CAN Talon SRX Ref"=w310) -> ()  [unwired: 7 in, 2 out]
        }
        frame Enabled {
          # "Up"
          # "Down"
          # "Pneumatic shooter code"
          # "Down"
          # "Up"
          n191 = Index Array(array=w326, index=2) -> (element=w325:dbl)
          n192 = Index Array(array=w329, index=4) -> (element=w321:bool)
          n193 = Greater Or Equal?(x=w325, y=0.75) -> (x >= y?=w323:bool)
          n194 = feedback #1(TRUE) -> (w315:bool)
          n195 = Not Or(1:w315, 2:w323) -> (0:w322:bool)
          n196 = Not Or(1:w322, 2:w321) -> (0:w314:bool)
          n197 = feedback-in #1(w314) -> ()
          n198 = Select(t=WPI_SolenoidValue."Off" ("Value"), s=w314, f=WPI_SolenoidValue."On") -> (s? t:f=w318:T6)
          n199 = call <vilib>:"WPI_SolenoidRefNum Registry Get.vi"("refnum name"="Shooter Lift") -> ("SolenoidDevRef"=w317:T20)  [unwired: 9 in, 1 out]
          n200 = call-poly <vilib>:"NT Write Value.vi"("Boolean"=w314, "Name"="Shooter up?") -> ()  [unwired: 9 in, 1 out]
          n201 = call-poly <vilib>:"WPI_SolenoidSet.vi"("Value"=w318, "SolenoidDevRef"=w317) -> ()  [unwired: 8 in, 2 out]
        }
      }
      n202 = call <vilib>:"WPI_MotorControlRefNum Registry Get.vi"("refnum name"="Right Driver 1") -> ("MotorControlDevRef"=w157:T10)  [unwired: 9 in, 1 out]
      n203 = call <vilib>:"WPI_MotorControlRefNum Registry Get.vi"("refnum name"="Right Driver 2") -> ("MotorControlDevRef"=w156:T10)  [unwired: 9 in, 1 out]
      n204 = call <vilib>:"WPI_MotorControlRefNum Registry Get.vi"("refnum name"="Left Driver 1") -> ("MotorControlDevRef"=w159:T10)  [unwired: 9 in, 1 out]
      n205 = call <vilib>:"WPI_MotorControlRefNum Registry Get.vi"("refnum name"="Left Driver 2") -> ("MotorControlDevRef"=w158:T10)  [unwired: 9 in, 1 out]
      n206 = Not(x=w138) -> (.not. x?=w137:bool)
      n207 = case shown="True" w137 {
        tunnel: w172 -> [_ w356]
        tunnel: w171 -> [_ w355]
        tunnel: w170 -> [_ w354]
        tunnel: w169 -> [_ w353]
        tunnel: w159 -> [w342 w352]
        tunnel: w158 -> [w343 w351]
        tunnel: w157 -> [w344 w350]
        tunnel: w156 -> [w341 w349]
        tunnel: w153 -> [w340 _]
        tunnel: [w338 w347] -> w99
        tunnel: [w337 w346] -> w98
        frame False {
          w345 = WPI_CANTalonSRX_APIControlMode."Percent VBus" ("Control Mode")
          n208 = Negate(x=w340) -> (-x=w339:dbl)
          n209 = call <vilib>:"WPI_CANTalonSRX_ChangeMode.vi"("Output"=w340, "Control Mode"=w345, "CAN Talon SRX Ref"=w342) -> ("CAN Talon SRX Ref"=w338:T10)  [unwired: 7 in, 1 out]
          n210 = call <vilib>:"WPI_CANTalonSRX_ChangeMode.vi"("Output"=w340, "Control Mode"=w345, "CAN Talon SRX Ref"=w343) -> ()  [unwired: 7 in, 2 out]
          n211 = call <vilib>:"WPI_CANTalonSRX_ChangeMode.vi"("Output"=w339, "Control Mode"=w345, "CAN Talon SRX Ref"=w344) -> ("CAN Talon SRX Ref"=w337:T10)  [unwired: 7 in, 1 out]
          n212 = call <vilib>:"WPI_CANTalonSRX_ChangeMode.vi"("Output"=w339, "Control Mode"=w345, "CAN Talon SRX Ref"=w341) -> ()  [unwired: 7 in, 2 out]
        }
        frame True {
          w348 = WPI_CANTalonSRX_APIControlMode."Percent VBus" ("Control Mode")
          n213 = call <vilib>:"WPI_CANTalonSRX_ChangeMode.vi"("Output"=w356, "Control Mode"=w348, "CAN Talon SRX Ref"=w352) -> ("CAN Talon SRX Ref"=w347:T10)  [unwired: 7 in, 1 out]
          n214 = call <vilib>:"WPI_CANTalonSRX_ChangeMode.vi"("Output"=w355, "Control Mode"=w348, "CAN Talon SRX Ref"=w351) -> ()  [unwired: 7 in, 2 out]
          n215 = call <vilib>:"WPI_CANTalonSRX_ChangeMode.vi"("Output"=w354, "Control Mode"=w348, "CAN Talon SRX Ref"=w350) -> ("CAN Talon SRX Ref"=w346:T10)  [unwired: 7 in, 1 out]
          n216 = call <vilib>:"WPI_CANTalonSRX_ChangeMode.vi"("Output"=w353, "Control Mode"=w348, "CAN Talon SRX Ref"=w349) -> ()  [unwired: 7 in, 2 out]
        }
      }
      n217 = call <vilib>:"WPI_CANTalonSRX_GetStatus.vi"("CAN Talon SRX Ref"=w98) -> ("Talon SRX Status"=w97:T17)  [unwired: 8 in, 2 out]
      n218 = call <vilib>:"WPI_CANTalonSRX_GetStatus.vi"("CAN Talon SRX Ref"=w99) -> ("Talon SRX Status"=w96:T17)  [unwired: 8 in, 2 out]
      n219 = Unbundle By Name(w96) -> ("Encoder Position"=→"left encoder":dbl)
      n220 = Unbundle By Name(w97) -> ("Encoder Position"=→"right encoder":dbl)
    }
  }
  n221 = Unbundle By Name("Match Info") -> ()  [unwired: 1 out]
  n222 = call <vilib>:"WPI_DriverStationReport Robot Code State.vi"("TeleOp"=TRUE ("Autonomous")) -> ()  [unwired: 10 in, 1 out]
  n223 = call <vilib>:"WPI_GyroRefNum Registry Get.vi"("refnum name"="Gyro") -> ("GyroDevRef"=w4:T7)  [unwired: 9 in, 1 out]
  n224 = call <vilib>:"WPI_GyroGetAngle.vi"("GyroDevRef"=w4) -> ("Angular Rate"=→"Angular Rate":dbl, "Angle"=w6:dbl)  [unwired: 6 in, 3 out]
  "Angle" <- w6
  n225 = call-poly <vilib>:"NT Write Value.vi"("Numeric"=w6, "Name"="gyro") -> ()  [unwired: 9 in, 1 out]
